vi "Main2.vi"() -> ()   [LabVIEW 2015]
uses:
  <vilib>/myRIO/Common/Instrument Driver Framework/myRIO v1.0/AI/vis/myRIO v1.1 Open AI.vi
  <vilib>/myRIO/Common/Instrument Driver Framework/myRIO v1.0/AI/vis/myRIO v1.2 Open AI.vi
  <vilib>/myRIO/Common/Instrument Driver Framework/roboRIO v1.0/AI/vis/roboRIO v1.0 Open AI.vi
  <vilib>/myRIO/Common/Instrument Driver Framework/myRIO v1.0/UART/vis/myRIO v1.0 Close UART.vi
  <vilib>/myRIO/Common/Instrument Driver Framework/Utilities/vis/Validate Channels.vi
  <vilib>/myRIO/Common/Instrument Driver Framework/myRIO v1.0/AI/vis/myRIO v1.0 Reserve AI.vi
  <vilib>/myRIO/Common/Instrument Driver Framework/roboRIO v1.0/AI/vis/roboRIO v1.0 Reserve AI.vi
  <vilib>/myRIO/Common/Instrument Driver Framework/myRIO v1.0/AI/vis/myRIO v1.0 Build MUX Configuration AI.vi
  <vilib>/myRIO/Common/Instrument Driver Framework/myRIO v1.0/Resource Manager/vis/myRIO v1.0 Reserve Channel List.vi
  <vilib>/myRIO/Common/Instrument Driver Framework/roboRIO v1.0/Resource Manager/vis/roboRIO v1.0 Reserve Channel List.vi
  <vilib>/myRIO/Common/Instrument Driver Framework/roboRIO v1.0/AI/vis/roboRIO v1.0 Build MUX Configuration AI.vi
  <vilib>/myRIO/Common/Instrument Driver Framework/myRIO v1.0/Resource Manager/vis/myRIO v1.0 Reserve Channel.vi
  <vilib>/myRIO/Common/Instrument Driver Framework/myRIO v1.0/Resource Manager/vis/myRIO v1.0 Unreserve Channel.vi
  <vilib>/myRIO/Common/Instrument Driver Framework/roboRIO v1.0/Resource Manager/vis/roboRIO v1.0 Reserve Channel.vi
  <vilib>/myRIO/Common/Instrument Driver Framework/roboRIO v1.0/Resource Manager/vis/roboRIO v1.0 Unreserve Channel.vi
  <vilib>/myRIO/Common/Instrument Driver Framework/myRIO v1.0/Resource Manager/vis/myRIO v1.0 Build Mutex Name.vi
  <vilib>/myRIO/Common/Instrument Driver Framework/roboRIO v1.0/Resource Manager/vis/roboRIO v1.0 Build Mutex Name.vi
  <vilib>/myRIO/Common/Instrument Driver Framework/Utilities/vis/Set_Get Target Info.vi
  <vilib>/Utility/error.llb/Error Cluster From Error Code.vi
  <vilib>/Utility/VariantDataType/GetNumericInfo.vi
  <vilib>/myRIO/Common/Instrument Driver Framework/myRIO v1.0/myRIO v1.1 Open.vi
  <vilib>/myRIO/Common/Instrument Driver Framework/myRIO v1.0/AI/vis/myRIO v1.0 Get Scaling Constants AI.vi
  <vilib>/myRIO/Common/Instrument Driver Framework/Utilities/vis/IO Manager.vi
  <vilib>/myRIO/Common/Instrument Driver Framework/Utilities/vis/Configuration Manager.vi
  <vilib>/myRIO/Common/Instrument Driver Framework/myRIO v1.0/myRIO v1.0 Close.vi
  <vilib>/myRIO/Common/Instrument Driver Framework/myRIO v1.0/myRIO v1.2 Open.vi
  <vilib>/myRIO/Common/Instrument Driver Framework/roboRIO v1.0/roboRIO v1.0 Open.vi
  <vilib>/myRIO/Common/Instrument Driver Framework/roboRIO v1.0/AI/vis/roboRIO v1.0 Get Scaling Constants AI.vi
  <vilib>/myRIO/Common/Instrument Driver Framework/myRIO v1.0/AI/vis/myRIO v1.0 Read AI.vi
  <vilib>/myRIO/Common/Instrument Driver Framework/roboRIO v1.0/AI/vis/roboRIO v1.0 Read AI.vi
  <vilib>/measure/mamon.llb/Waveform Peak Detection for 1 Chan.vi
  <vilib>/myRIO/Common/Instrument Driver Framework/Utilities/vis/FPGA Ref Manager.vi
  <vilib>/myRIO/Common/Instrument Driver Framework/myRIO v1.0/myRIO v1.0 Reset FPGA.vi
  <vilib>/myRIO/Common/Instrument Driver Framework/myRIO v1.0/IRQ/vis/myRIO v1.0 IRQ Info FGV.vi
  <vilib>/myRIO/Common/Instrument Driver Framework/myRIO v1.0/IRQ/vis/myRIO v1.0 Timer IRQ Info FGV.vi
  <vilib>/myRIO/Instrument Drivers/Utilities/Utilities.lvlib
  <vilib>/myRIO/Instrument Drivers/Onboard IO/AI/AI.lvlib
  <vilib>/measure/NI_MAPro.lvlib
panel:
  out "x-y 2":dbl[](array[numeric])
  out "x-y":dbl[](array[numeric])
  in  "threshold 2":dbl format="%.2p"
  in  "threshold":dbl format="%.2p"
  out "Amplitudes 2":dbl[](array[numeric]) format="%.2p"
  out "Amplitudes":dbl[](array[numeric]) format="%.2p"
  # "right-click when stopped to adjust\nchart history length from the default\nvalue of 1024"
  # "Electret microphone demo"
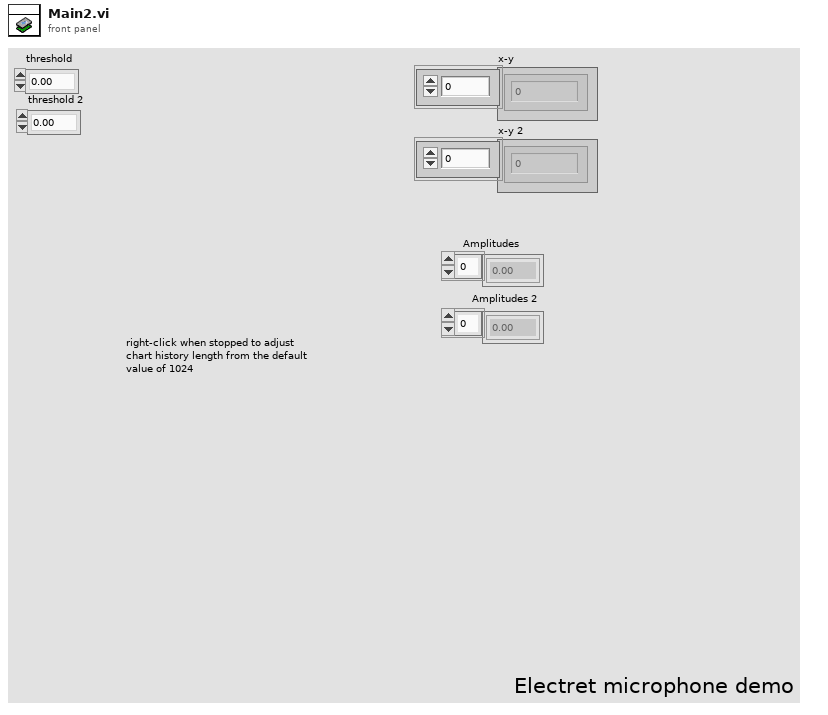
[diagram p1: front panel]
types:
  T1 = typedef "AI.lvlib/AI Reference.ctl" = cluster{"myRIO Reference":T2, "AI Channels List":T6, "AI Scaling Constants List":T8}
  T2 = typedef "myRIO Generic Hardware Reference.ctl" = cluster{"myRIO Model":T3, "myRIO Hardware Reference":T4}
  T3 = typedef "Hardware Version Enum.ctl" = enum16{"Unknown", "myRIO-1900", "myRIO-1950", "roboRIO"}
  T4 = typedef "myRIO v1.0 Reference.ctl" = cluster{"Generic FPGA Reference":T5, "Allow multiple opens":bool}
  T5 = typedef "Generic FPGA Reference.ctl" = refnum<k20>
  T6 = typedef "AI Channels List.ctl" = T7[]
  T7 = typedef "AI Channels Enum.ctl" = enum16{"Not Connected", "AudioIn/Left", "AudioIn/Right", "C/AI0", "C/AI1", "A/AI0", "A/AI1", "A/AI2", "A/AI3", "B/AI0", "B/AI1", "B/AI2", "B/AI3", "AI/AI0", "AI/AI1", "AI/AI2", "AI/AI3"}
  T8 = typedef "Analog Scaling Constants List.ctl" = T9[]
  T9 = typedef "Analog Scaling Constants.ctl" = cluster{"LSB Weight (Volts)":dbl, "Offset (Volts)":dbl, "Signed?":bool}
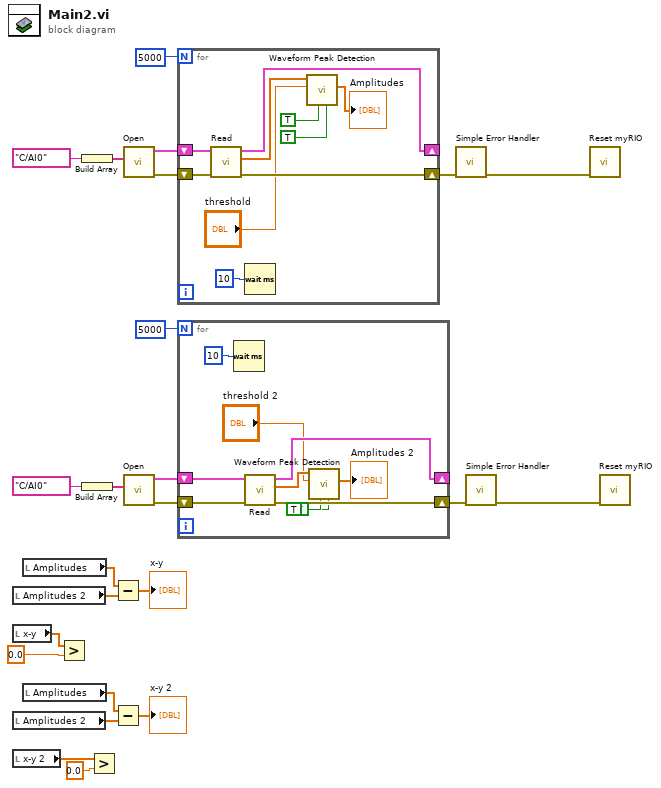
[diagram p0: block diagram]
diagram:
  n1 = local read "Amplitudes 2"() -> (w9:dbl[])
  n2 = local read "x-y"() -> (w4:dbl[])
  n3 = local read "Amplitudes 2"() -> (w6:dbl[])
  n4 = local read "x-y 2"() -> (w2:dbl[])
  n5 = local read "Amplitudes"() -> (w10:dbl[])
  n6 = local read "Amplitudes"() -> (w7:dbl[])
  n7 = Greater?(x=w4, y=0.0) -> ()  [unwired: 1 out]
  n8 = Build Array(tag "C/AI0" ("myRIO AI Channel")) -> (w23:tag[])
  n9 = Build Array(tag "C/AI0" ("myRIO AI Channel")) -> (w16:tag[])
  n10 = Greater?(x=w2, y=0.0) -> ()  [unwired: 1 out]
  n11 = Subtract(x=w10, y=w9) -> (x-y=→"x-y":dbl[])
  n12 = Subtract(x=w7, y=w6) -> (x-y=→"x-y 2":dbl[])
  n13 = call <vilib>:"Open.vi"("Channel Names"=w23) -> ("error out"=w21:errorcluster, "AI Ref Out"=w22:T1)  [unwired: 9 in]
  n14 = call <vilib>:"Open.vi"("Channel Names"=w16) -> ("error out"=w14:errorcluster, "AI Ref Out"=w15:T1)  [unwired: 9 in]
  n15 = for {
    N: 5000 -> [_]
    shift-right: [w30] -> _
    shift-left: w22 -> [w33]
    shift-right: [w31] -> w19
    shift-left: w21 -> [w34]
    n16 = call <vilib>:"Read.vi"("error in (no error)"=w34, "AI Ref In"=w33) -> ("error out"=w31:errorcluster, "Values"=w29:dbl[], "AI Ref Out"=w30:T1)  [unwired: 7 in]
    n17 = Wait (ms)(milliseconds to wait=u32 10) -> ()  [unwired: 1 out]
    n18 = call-poly <vilib>:"Waveform Peak Detection.vi"("end of data (T)"=TRUE, "initialize (T)"=TRUE, "threshold"="threshold", "Signal In"=w29) -> ("Amplitudes"=→"Amplitudes":dbl[])  [unwired: 3 in, 4 out]
  }
  n19 = for {
    N: 5000 -> [_]
    shift-right: [w42] -> _
    shift-left: w15 -> [w43]
    shift-right: [w40] -> w12
    shift-left: w14 -> [w44]
    n20 = Wait (ms)(milliseconds to wait=u32 10) -> ()  [unwired: 1 out]
    n21 = call <vilib>:"Read.vi"("error in (no error)"=w44, "AI Ref In"=w43) -> ("error out"=w40:errorcluster, "Values"=w39:dbl[], "AI Ref Out"=w42:T1)  [unwired: 7 in]
    n22 = call-poly <vilib>:"Waveform Peak Detection.vi"("end of data (T)"=TRUE, "initialize (T)"=TRUE, "threshold"="threshold 2", "Signal In"=w39) -> ("Amplitudes"=→"Amplitudes 2":dbl[])  [unwired: 3 in, 4 out]
  }
  n23 = call <vilib>:"Simple Error Handler.vi"("error in (no error)"=w19) -> ("error out"=w20:errorcluster)  [unwired: 4 in, 4 out]
  n24 = call <vilib>:"Simple Error Handler.vi"("error in (no error)"=w12) -> ("error out"=w13:errorcluster)  [unwired: 4 in, 4 out]
  n25 = call <vilib>:"Reset myRIO.vi"("error in (no error)"=w20) -> ()  [unwired: 10 in, 1 out]
  n26 = call <vilib>:"Reset myRIO.vi"("error in (no error)"=w13) -> ()  [unwired: 10 in, 1 out]
